vi "TDMS Read Events Data.vi"() -> ()   [LabVIEW 2023]
doc: "This example demonstrates how to read measured data, text and timestamps from a .tdms file using the TDMS API."
panel:
  out "Measured Data":waveform(dbl)[](graph)
  in  "Event Data":i32(listbox)=-1
  # "Overview: Demonstrates the use of the TDMS Read function to read measured data, text and timestamps from an existing .tdms file.\nInstructions:\n1. Make sure you have already run TDMS Write Events Data.vi.\n2. Run this VI.\n3. Delete the .tdms file (located at [LabVIEW Data]\\Example Events Data.tdms) when you are done."
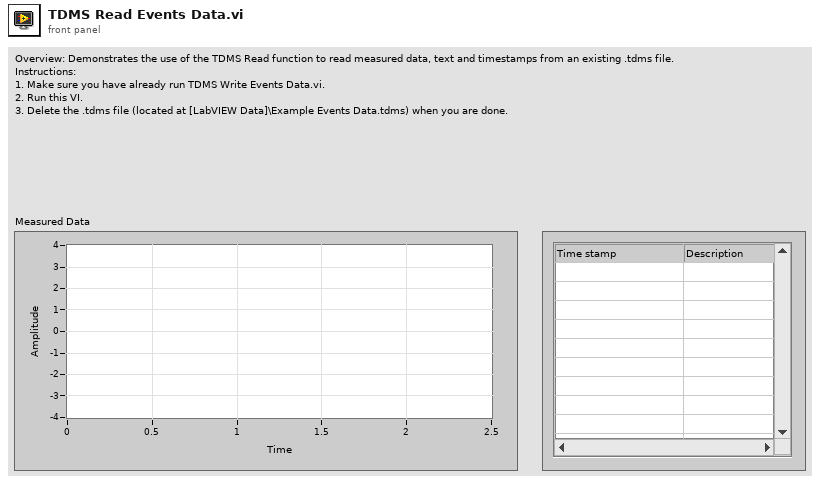
[diagram p1: front panel]
types:
  T1 = enum16{"open", "open or create", "create or replace", "create", "open (read-only)"}
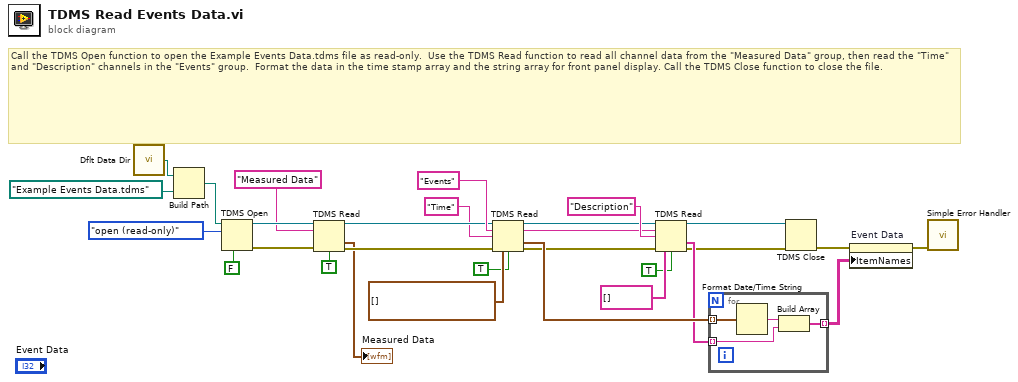
[diagram p0: block diagram]
diagram:
  # "Call the TDMS Open function to open the Example Events Data.tdms file as read-only.  Use the TDMS Read function to read all channel data from the \"Measured Data\" group, then read the \"Time\" and \"Description\" channels in the \"Events\" group.  Format the data in the time stamp array and the string array for front panel display. Call the TDMS Close function to close the file."
  n1 = call <vilib>:"Dflt Data Dir.vi"() -> ("App:Default Data Directory"=w29:path)
  n2 = Build Path(base path=w29, name or relative path=path "Example Events Data.tdms" ("file path")) -> (appended path=w12:path)
  n3 = TDMS Open(6:FALSE ("disable buffering (T)"), 10:T1."open (read-only)" ("operation"), 11:w12) -> (0:w25:errorcluster, 3:w26:refnum<k34>)  [unwired: 4 in]
  n4 = TDMS Read(0:w26, 5:"Measured Data" ("group name"), 11:w25, 13:TRUE ("return channels in file order? (F)")) -> (4:w22:refnum<k34>, 10:→"Measured Data":waveform(dbl)[], 15:w8:errorcluster)  [unwired: 4 in, 3 out]
  n5 = TDMS Read(0:w22, 5:"Events", 7:"Time", 11:w8, 12:timestamp[] [], 13:TRUE ("return channels in file order? (F)")) -> (4:w18:refnum<k34>, 6:w15:string, 10:w14:timestamp[], 15:w7:errorcluster)  [unwired: 2 in, 2 out]
  n6 = TDMS Read(0:w18, 5:w15, 7:"Description", 11:w7, 12:string[] [], 13:TRUE ("return channels in file order? (F)")) -> (4:w17:refnum<k34>, 10:w13:string[], 15:w6:errorcluster)  [unwired: 2 in, 3 out]
  n7 = for {
    tunnel: w14 -> [w33] mode=indexing
    tunnel: w13 -> [w31] mode=indexing
    tunnel: [w30] -> w4 mode=indexing
    n8 = Format Date/Time String(seconds (now)=w33) -> (date/time string=w32:string)  [unwired: 2 out]
    n9 = Build Array(w32, w31) -> (w30:string[])
  }
  n10 = TDMS Close(8:w6, 11:w17) -> (0:w3:errorcluster)  [unwired: 1 out]
  n11 = property on="Event Data" class="MCListbox (strict)"(error in=w3, "ItemNames"=w4) -> (error out=w2:errorcluster)  [unwired: 1 in, 1 out]
  n12 = call <vilib>:"Simple Error Handler.vi"("error in (no error)"=w2) -> ()  [unwired: 1 in, 8 out]
